vi "main_subvi_pattern_2.vi"(0 "Refnum Original Bild":T1, 1 "Länge der Spur":i32, 2 "Parameters Pattern":T3, 3 "Länge des Pfeils":sgl, 4 "Object Tracking Session Out in":T2, 5 "Refnum Tracking":T1, 6 "Array in":dbl[][](array[numeric]), 7 "Minimum Score":i32, 8 "Mittelpunktgröße":sgl, 9 "Numeric 2":i32, 10 "Pattern1 Farbe":u32, 11 "Numeric":i32, 12 "Image Matching":T1, 13 "Template Image In":T1) -> (14 "Refnum OUt":T1, 15 "Array out":dbl[][](array[numeric]), 16 "Object Tracking Session Out out":T2, 17 "String":string)   [LabVIEW 2014]
uses:
  <vilib>/vision/Image Controls.llb/IMAQ Image.ctl
  <vilib>/vision/Tracking.llb/IMAQ Object Tracking Session.ctl
  <vilib>/vision/NI_Vision_Development_Module.lvlib
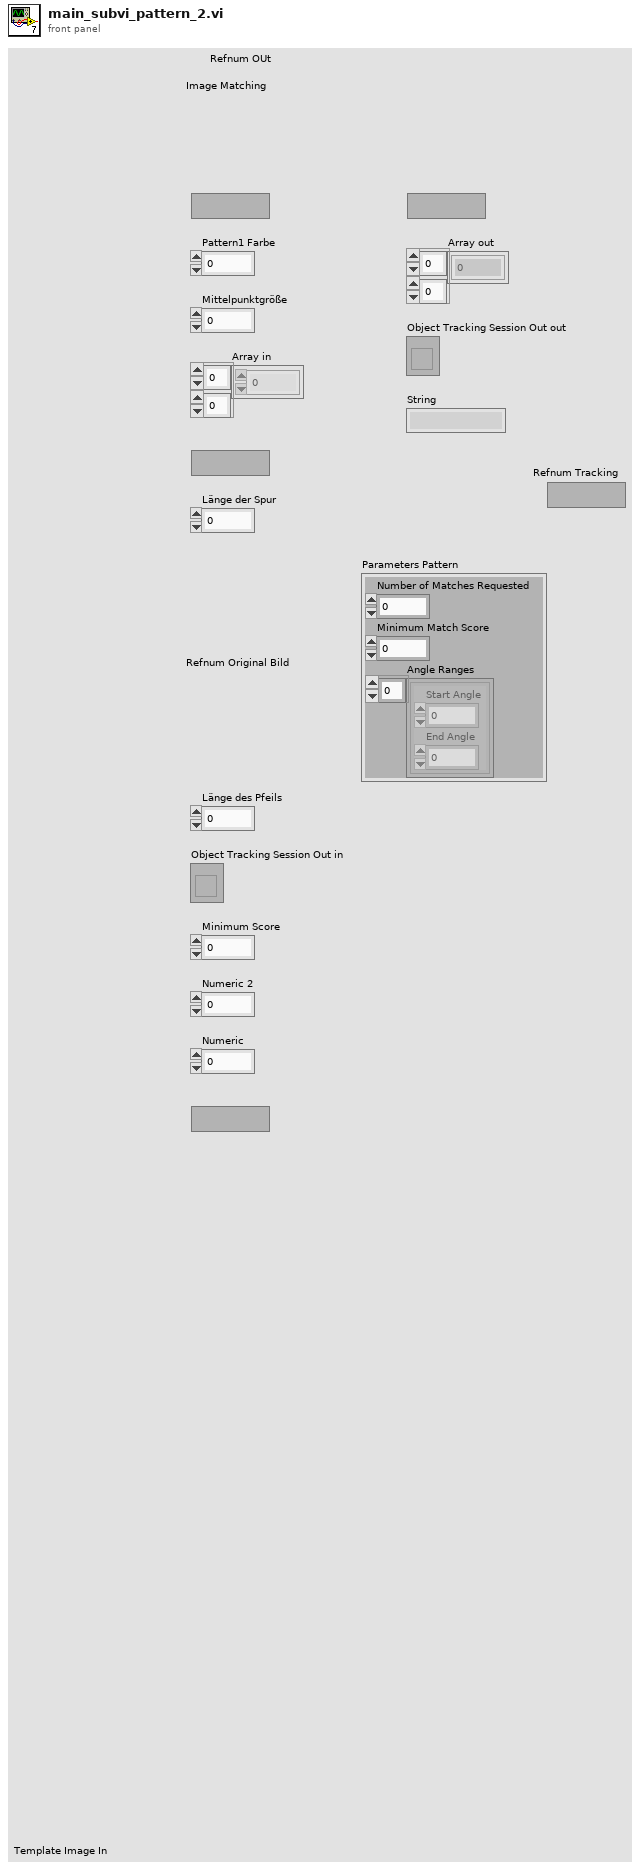
[diagram p1: front panel]
types:
  T1 = typedef "IMAQ Image.ctl" = refnum<image>
  T2 = typedef "IMAQ Object Tracking Session.ctl" = refnum<k20>
  T3 = cluster{"Number of Matches Requested":i32, "Minimum Match Score":sgl, "Angle Ranges":cluster{"Start Angle":sgl, "End Angle":sgl}[]}
  T4 = cluster{"Position":cluster{"x":sgl, "y":sgl}, "Angle":sgl, "Scale":sgl, "Score":sgl, "Bounding Box":cluster{"x":sgl, "y":sgl}[]}[]
  T5 = typedef "Image Type" = u32
  T6 = typedef "ROI Descriptor" = cluster{"Global Rectangle":i32[], "Contours":cluster{"ID":enum32{"External", "Internal"}, "Type":u32, "Coordinates":i32[]}[]}
  T7 = cluster{"Label":string, "Score":i32, "Angle":dbl, "Location":cluster{"X":dbl, "Y":dbl}, "Bounding Box":cluster{"X":dbl, "Y":dbl}[], "Object Found?":bool}[]
  T8 = cluster{"Label":string, "Score":i32, "Angle":dbl, "Location":cluster{"X":dbl, "Y":dbl}, "Bounding Box":cluster{"X":dbl, "Y":dbl}[], "Object Found?":bool}
  T9 = cluster{"Matches (pixel)[0]":cluster{"Position":cluster{"x":sgl, "y":sgl}, "Angle":sgl, "Scale":sgl, "Score":sgl, "Bounding Box":cluster{"x":sgl, "y":sgl}[]}, "Matches (pixel)[1]":cluster{"Position":cluster{"x":sgl, "y":sgl}, "Angle":sgl, "Scale":sgl, "Score":sgl, "Bounding Box":cluster{"x":sgl, "y":sgl}[]}, "Matches (pixel)[2]":cluster{"Position":cluster{"x":sgl, "y":sgl}, "Angle":sgl, "Scale":sgl, "Score":sgl, "Bounding Box":cluster{"x":sgl, "y":sgl}[]}, "Matches (pixel)[3]":cluster{"Position":cluster{"x":sgl, "y":sgl}, "Angle":sgl, "Scale":sgl, "Score":sgl, "Bounding Box":cluster{"x":sgl, "y":sgl}[]}, "Matches (pixel)[4]":cluster{"Position":cluster{"x":sgl, "y":sgl}, "Angle":sgl, "Scale":sgl, "Score":sgl, "Bounding Box":cluster{"x":sgl, "y":sgl}[]}, "Matches (pixel)[5]":cluster{"Position":cluster{"x":sgl, "y":sgl}, "Angle":sgl, "Scale":sgl, "Score":sgl, "Bounding Box":cluster{"x":sgl, "y":sgl}[]}, "Matches (pixel)[6]":cluster{"Position":cluster{"x":sgl, "y":sgl}, "Angle":sgl, "Scale":sgl, "Score":sgl, "Bounding Box":cluster{"x":sgl, "y":sgl}[]}, "Matches (pixel)[7]":cluster{"Position":cluster{"x":sgl, "y":sgl}, "Angle":sgl, "Scale":sgl, "Score":sgl, "Bounding Box":cluster{"x":sgl, "y":sgl}[]}, "Matches (pixel)[8]":cluster{"Position":cluster{"x":sgl, "y":sgl}, "Angle":sgl, "Scale":sgl, "Score":sgl, "Bounding Box":cluster{"x":sgl, "y":sgl}[]}}
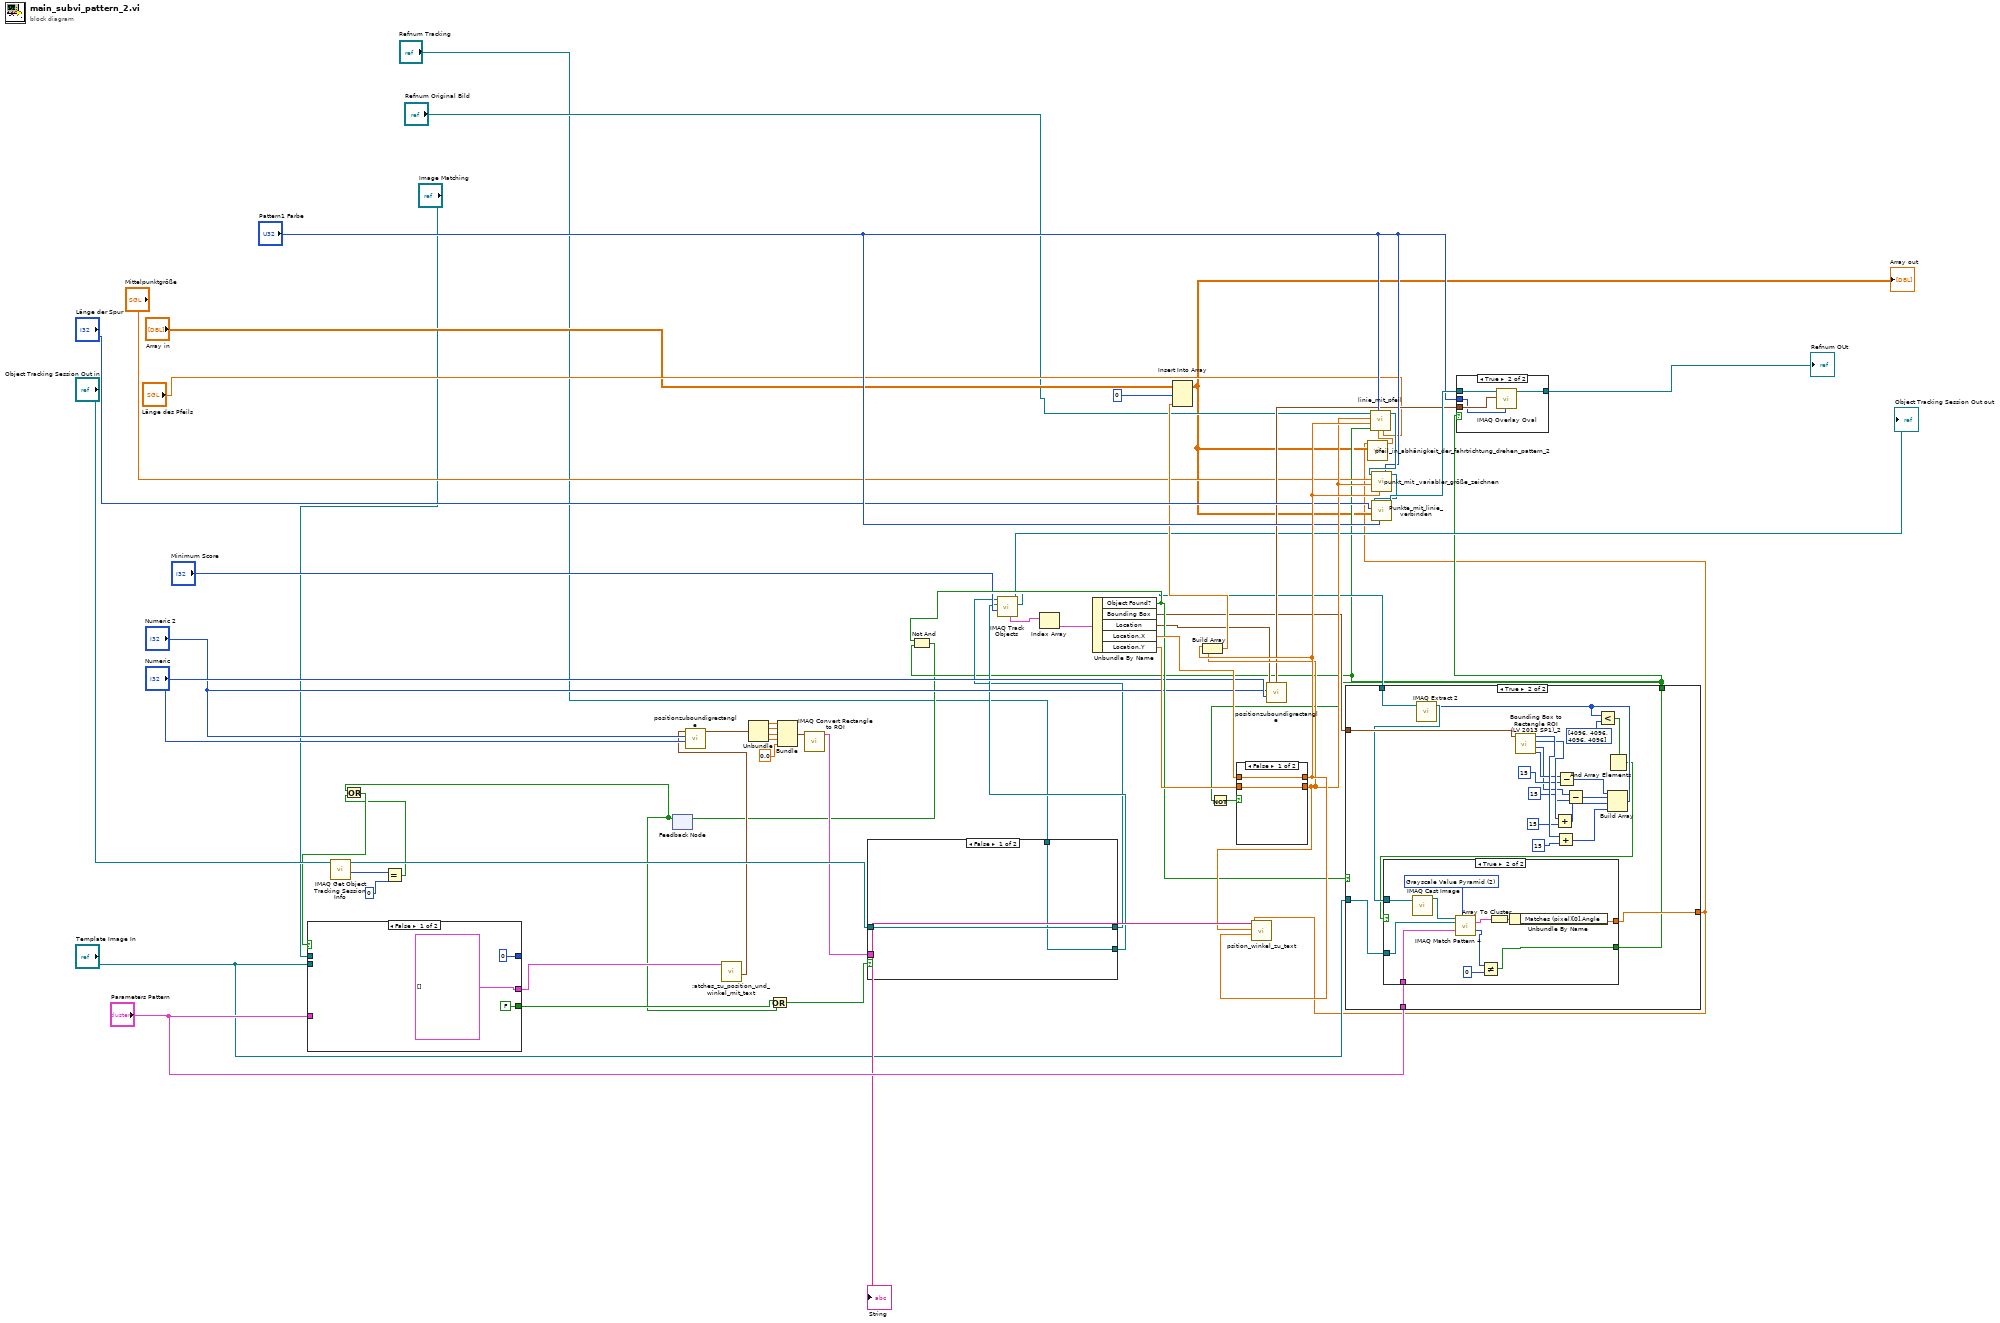
[diagram p0: block diagram]
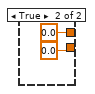
[diagram p2: hidden frame]
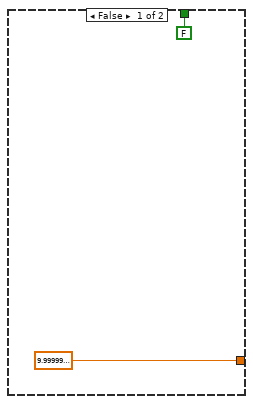
[diagram p3: hidden frame]
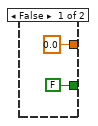
[diagram p4: hidden frame]
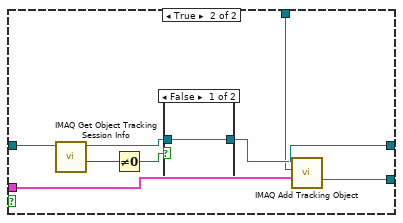
[diagram p5: hidden frame]
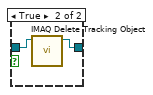
[diagram p6: hidden frame]
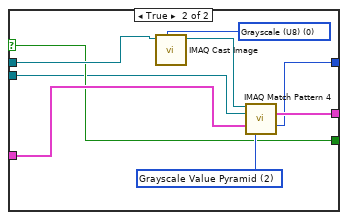
[diagram p7: hidden frame]
diagram:
  n1 = call "IMAQ Get Object Tracking Session Info"("Object Tracking Session In"="Object Tracking Session Out in") -> ("Number of Objects"=w47:i32, "Object Tracking Session Out"=w46:T2)  [unwired: 7 in, 2 out]
  n2 = Equal?(x=w47, y=0) -> (x = y?=w6:bool)
  n3 = feedback #1() -> (w7:bool)  [unwired: 1 in]
  n4 = Or(x=w7, y=w6) -> (x .or. y?=w41:bool)
  n5 = case shown="False" w41 {
    selector: w41 -> [_ w64]
    tunnel: [0 ("Number of Matches (Pattern Matching 1)") w69] -> _
    tunnel: "Image Matching" -> [_ w67]
    tunnel: [T4 [] ("Matches (Pattern Matching 1)") w70] -> w18
    tunnel: "Parameters Pattern" -> [_ w71]
    tunnel: "Template Image In" -> [_ w63]
    tunnel: [FALSE w64] -> w11
    frame False {
    }
    frame True {
      w65 = T5 0 items=["Grayscale (U8)", "Grayscale (I16)", "Grayscale (SGL)", "Complex (CSG)", "RGB (U32)", "HSL (U32)", "RGB (U64)", "Grayscale (U16)"] ("Image Type")
      w68 = 2 items=["All", "Low Discrepancy Sampling", "Grayscale Value Pyramid", "Gradients Pyramid"] ("Algorithm")
      n6 = call "IMAQ Cast Image"("Image Type"=w65, "Image Src"=w67) -> ("Image Dst Out"=w66:T1)  [unwired: 8 in, 1 out]
      n7 = call "IMAQ Match Pattern 4"("Image"=w66, "Algorithm"=w68, "Template Image"=w63, "Parameters"=w71) -> ("Matches (pixel)"=w70:T4, "Number of Matches"=w69:i32)  [unwired: 7 in, 3 out]
    }
  }
  n8 = call ";atches_zu_position_und_winkel_mit_text.vi"("Matches (Pattern Matching 1)"=w18) -> ("Position"=w17:cluster{"x":sgl, "y":sgl})  [unwired: 3 in, 7 out]
  n9 = call "positionzuboundigrectangle.vi"("Y Resolution"="Numeric", "X Resolution"="Numeric 2", "Position"=w17) -> ("Cluster"=w21:cluster{dbl, dbl, dbl, dbl})  [unwired: 8 in]
  n10 = Unbundle(w21) -> (w22:dbl, w23:dbl, w24:dbl, w25:dbl)
  n11 = Or(x=w11, y=w7) -> (x .or. y?=w12:bool)
  n12 = Bundle(w22, w23, w24, w25, "y"=0.0) -> (w27:cluster{dbl, dbl, dbl, dbl, "y":dbl})  [unwired: 1 in]
  n13 = call "IMAQ Convert Rectangle to ROI"("Rectangle"=w27) -> ("ROI Descriptor"=w28:T6)  [unwired: 8 in, 1 out]
  n14 = case shown="False" w12 {
    tunnel: w28 -> [_ w82]
    tunnel: [w73 w81] -> w29
    tunnel: [w72 w80] -> w30
    tunnel: w46 -> [w73 w78]
    tunnel: "Refnum Tracking" -> [w72 w74]
    frame False {
    }
    frame True {
      n15 = call "IMAQ Get Object Tracking Session Info"("Object Tracking Session In"=w78) -> ("Number of Objects"=w79:i32, "Object Tracking Session Out"=w77:T2)  [unwired: 7 in, 2 out]
      n16 = Not Equal To 0?(x=w79) -> (x != 0?=w76:bool)
      n17 = case shown="False" w76 {
        tunnel: [w83 w85] -> w75
        tunnel: w77 -> [w83 w84]
        frame False {
        }
        frame True {
          n18 = call "IMAQ Delete Tracking Object"("Object Tracking Session In"=w84) -> ("Object Tracking Session Out"=w85:T2)  [unwired: 9 in, 1 out]
        }
      }
      n19 = call "IMAQ Add Tracking Object"("ROI Descriptor"=w82, "Image"=w74, "Object Tracking Session In"=w75) -> ("Image (duplicate)"=w80:T1, "Object Tracking Session Out"=w81:T2)  [unwired: 6 in, 1 out]
    }
  }
  n20 = call "IMAQ Track Objects"("Minimum Score"="Minimum Score", "Image"=w30, "Object Tracking Session In"=w29) -> ("Image (duplicate)"=w34:T1, "Object Tracking Session Out"=→"Object Tracking Session Out out":T2, "Objects (real-world)"=w55:T7)  [unwired: 4 in, 2 out]
  n21 = Index Array(array=w55) -> (element=w31:T8)  [unwired: 1 in]
  n22 = Unbundle By Name(w31) -> ("Object Found?"=w42:bool, "Bounding Box"=w35:cluster{"X":dbl, "Y":dbl}[], "Location"=w36:cluster{"X":dbl, "Y":dbl}, "Location.X"=w43:dbl, "Location.Y"=w44:dbl)
  n23 = call "positionzuboundigrectangle.vi"("Y Resolution"="Numeric", "X Resolution"="Numeric 2", "Position"=w36) -> ("Cluster"=w39:cluster{dbl, dbl, dbl, dbl})  [unwired: 8 in]
  n24 = case shown="True" w42 {
    tunnel: "Template Image In" -> [_ w110]
    tunnel: [sgl 1e+23 ("Angle") w109] -> w2
    tunnel: "Parameters Pattern" -> [_ w108]
    tunnel: w34 -> [_ w95]
    tunnel: w35 -> [_ w94]
    tunnel: [FALSE w93] -> w13
    frame False {
    }
    frame True {
      n25 = call "Bounding Box to Rectangle ROI (LV 2013 SP1)_2.vi"("Bounding Box"=w94) -> ("Left"=w99:i16, "Top"=w96:i16, "Right"=w102:i16, "Bottom"=w106:i16)  [unwired: 7 in]
      n26 = Add(x=w102, y=i16 15) -> (x+y=w104:i16)
      n27 = Add(x=w106, y=i16 15) -> (x+y=w107:i16)
      n28 = Subtract(x=w99, y=i16 15) -> (x-y=w101:i16)
      n29 = Subtract(x=w96, y=i16 15) -> (x-y=w97:i16)
      n30 = Build Array(w101, w97, w104, w107) -> (w91:i16[])
      n31 = call "IMAQ Extract 2"("Optional Rectangle"=w91, "Image Src"=w95) -> ("Image Dst Out"=w92:T1)  [unwired: 8 in, 1 out]
      n32 = Less?(x=w91, y=i16[] [4096, 4096, 4096, 4096]) -> (x < y?=w89:bool[])
      n33 = And Array Elements(Boolean array=w89) -> (logical AND=w88:bool)
      n34 = case shown="True" w88 {
        tunnel: w110 -> [_ w122]
        tunnel: [sgl 0.0 ("Angle") w119] -> w109
        tunnel: w108 -> [_ w118]
        tunnel: [FALSE w115] -> w93
        tunnel: w92 -> [_ w114]
        frame False {
        }
        frame True {
          w123 = 2 items=["All", "Low Discrepancy Sampling", "Grayscale Value Pyramid", "Gradients Pyramid"] ("Algorithm")
          n35 = call "IMAQ Cast Image"("Image Src"=w114) -> ("Image Dst Out"=w113:T1)  [unwired: 9 in, 1 out]
          n36 = call "IMAQ Match Pattern 4"("Image"=w113, "Algorithm"=w123, "Template Image"=w122, "Parameters"=w118) -> ("Matches (pixel)"=w121:T4, "Number of Matches"=w117:i32)  [unwired: 7 in, 3 out]
          n37 = Not Equal?(x=w117, y=0) -> (x != y?=w115:bool)
          n38 = Array To Cluster(array=w121) -> (cluster=w120:T9)
          n39 = Unbundle By Name(w120) -> ("Matches (pixel)[0].Angle"=w119:sgl)
        }
      }
    }
  }
  n40 = Not And(1:w13, 2:w42) -> (0:w8:bool)
  n41 = feedback-in #1(w8) -> ()
  n42 = Not(x=w13) -> (.not. x?=w14:bool)
  n43 = case shown="False" w14 {
    tunnel: w43 -> [w125 _]
    tunnel: w44 -> [w124 _]
    tunnel: [w125 0.0 ("X")] -> w57
    tunnel: [w124 0.0 ("Y")] -> w56
    frame False {
    }
    frame True {
    }
  }
  n44 = Build Array(w57, w56) -> (w40:dbl[])
  n45 = Insert Into Array "Insert Into Array"(array="Array in", index (row)=0 ("index"), new element=w40) -> (w3:dbl[][])  [unwired: 1 in]
  "Array out" <- w3
  n46 = call "psition_winkel_zu_text.vi"("X"=w57, "Y"=w56, "Angle"=w2) -> ("String"=→"String":string)  [unwired: 8 in]
  n47 = call "pfeil_in_abhänigkeit_der_fahrtrichtung_drehen_pattern_2.vi"("Array"=w3, "Angle in"=w2) -> ("Angle out"=w1:sgl)  [unwired: 9 in]
  n48 = call "linie_mit_pfeil.vi"("Richtungspfeillänge"="Länge des Pfeils", "Angle"=w1, "Color"="Pattern1 Farbe", "Boolean"=w13, "x"=w57, "y"=w56, "Refnum in"="Refnum Original Bild") -> ("Refnum out"=w51:T1)  [unwired: 4 in]
  n49 = call "punkt_mit _variabler_größe_zeichnen.vi"("Color"="Pattern1 Farbe", "x"=w57, "y"=w56, "größe"="Mittelpunktgröße", "Refnum in"=w51) -> ("Refnum out"=w52:T1)  [unwired: 5 in, 1 out]
  n50 = call "Punkte_mit_linie_verbinden.vi"("Color"="Pattern1 Farbe", "Array"=w3, "dimension size"="Länge der Spur", "Refnum in"=w52) -> ("Refnum out"=w53:T1)  [unwired: 7 in]
  n51 = case shown="True" w13 {
    tunnel: w39 -> [_ w132]
    tunnel: [w128 w131] -> w54
    tunnel: w53 -> [w128 w130]
    tunnel: "Pattern1 Farbe" -> [_ w129]
    frame False {
    }
    frame True {
      n52 = call "IMAQ Overlay Oval"("Color"=w129, "Bounding Rectangle"=w132, "Image"=w130) -> ("Image Out"=w131:T1)  [unwired: 7 in, 1 out]
    }
  }
  "Refnum OUt" <- w54
